vi "LAN Trigger Connect.vi"(8 "error in":errorcluster, 9 "Trigger # (1)":u32=1 min=1 max=8, 10 "Node In":string, 11 "VISA resource name":refnum<visa-resource-name>) -> (0 "error out":errorcluster, 2 "Node Out":string, 3 "VISA resource name out":refnum<visa-resource-name>, 4 "Command String":string)   [LabVIEW 2018, in "Keithley 2600 Series.lvlib"]
doc: "This VI connects the selected LAN trigger.\n\n<b>Remarks:</b>\nCall Config LAN Trigger.vi prior to this VI to configure the trigger. This VI does not check to see if connection was successful. Call LAN Trigger Connected.vi to check LAN trigger connection status.\n\n<b>Functions and Attributes Used</b>\nlan.trigger[n].connect()"
uses:
  Keithley 2600 Series.lvlib
panel:
  # "(c) 2008 Keithley Instruments, Inc.  ALL RIGHTS RESERVED."
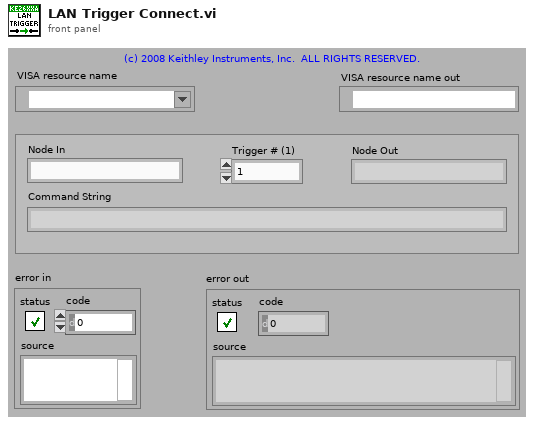
[diagram p1: front panel]
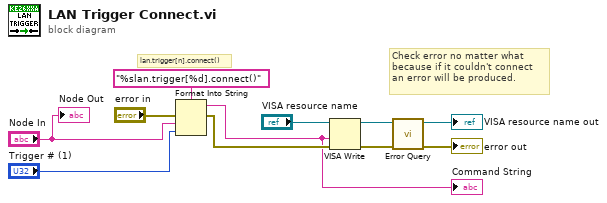
[diagram p0: block diagram]
diagram:
  # "Check error no matter what\nbecause if it couldn't connect\nan error will be produced."
  # "lan.trigger[n].connect()"
  n1 = Format Into String(format string="%slan.trigger[%d].connect()", error in="error in", "Node In", "Trigger # (1)") -> (resulting string=w1:string, error out=w7:errorcluster)  [unwired: 1 in]
  "Command String" <- w1
  n2 = VISA Write(VISA resource name="VISA resource name", write buffer=w1, error in (no error)=w7) -> (VISA resource name out=w5:refnum<visa-resource-name>, error out=w4:errorcluster)  [unwired: 1 out]
  n3 = call "Error Query.vi"("error in (no error)"=w4, "VISA resource name"=w5) -> ("error out"=→"error out":errorcluster, "VISA resource name out"=→"VISA resource name out":refnum<visa-resource-name>)  [unwired: 8 out]
  "Node Out" <- "Node In"
